vi "Get extension from URL.vi"(11 "url":string) -> (3 "Extension":string)   [LabVIEW 2010]
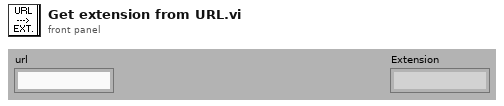
[diagram p1: front panel]
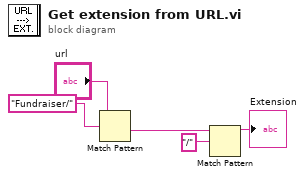
[diagram p0: block diagram]
diagram:
  n1 = Match Pattern(string="url", regular expression="Fundraiser/") -> (after substring=w4:string)  [unwired: 1 in, 3 out]
  n2 = Match Pattern(string=w4, regular expression="/") -> (before substring=→"Extension":string)  [unwired: 1 in, 3 out]
